vi "个人信息查询跳出界面.vi"() -> (11 "Boolean":bool)   [LabVIEW 2023]
uses:
  <vilib>/Utility/file.llb/Read From Spreadsheet File (string).vi
panel:
  in  "信息查询":i32(listbox)
  in  "输入选项":i32(ring) items=["姓名", "学号", "寝室号"]
  out "Array":string[][](array[string])
  in  "确认":bool
  in  "退出":bool
  in  "姓名/学号/寝室号":string
  # "个人信息查询"
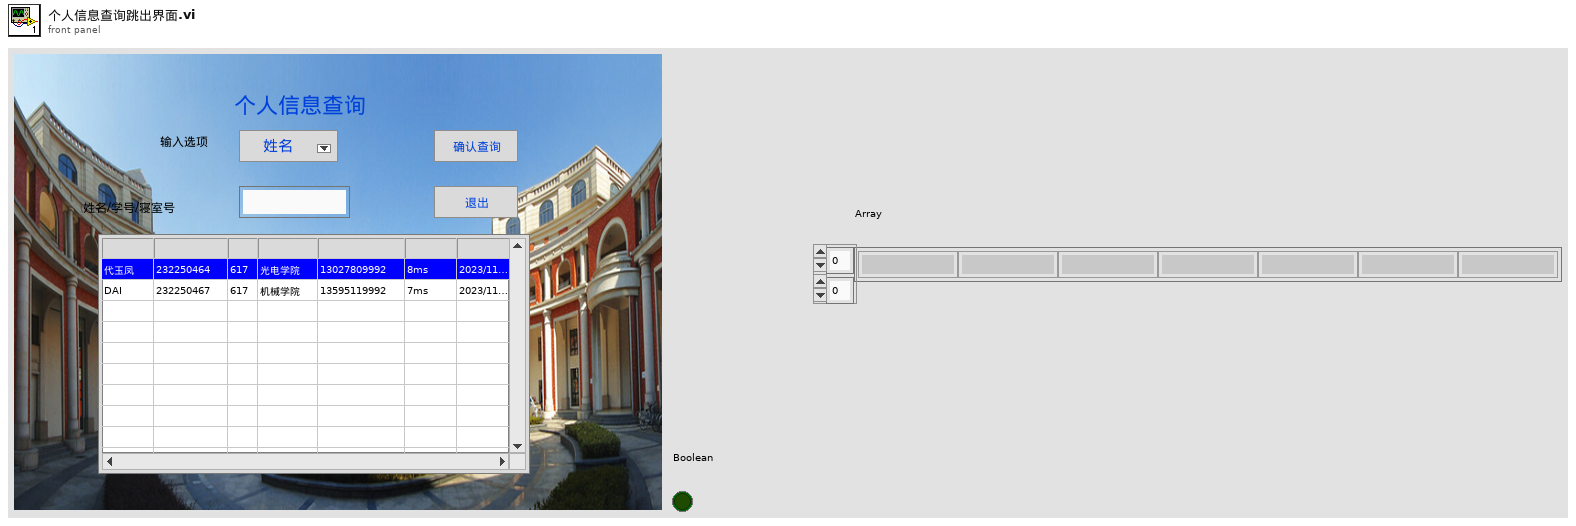
[diagram p1: front panel]
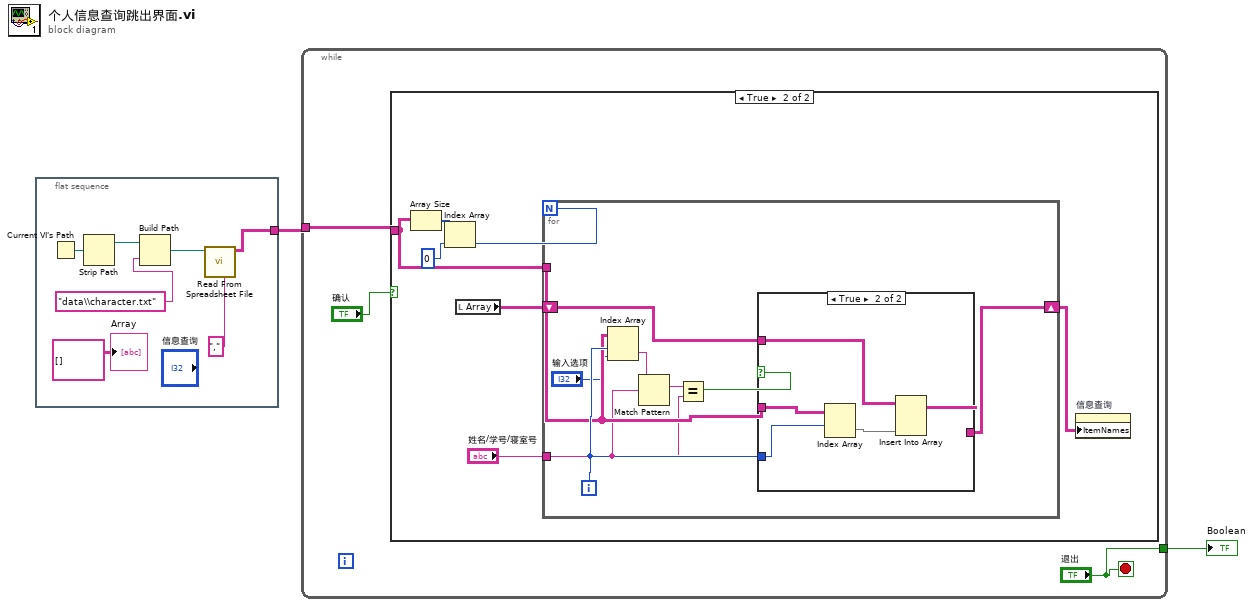
[diagram p0: block diagram]
diagram:
  n1 = flat-sequence {
    tunnel: [w4] -> w2
    frame #0 {
      n2 = Current VI's Path() -> (path=w7:path)
      n3 = Strip Path(path=w7) -> (stripped path=w9:path)  [unwired: 1 out]
      n4 = Build Path(base path=w9, name or relative path="data\\character.txt") -> (appended path=w8:path)
      n5 = call-poly <vilib>:"Read From Spreadsheet File.vi"("delimiter (\\t)"=",", "file path (dialog if empty)"=w8) -> ("all rows"=w4:string[][])  [unwired: 5 in, 4 out]
      "Array" <- string[][] [] ("Array")
    }
  }
  n6 = while {
    tunnel: w2 -> [w11]
    tunnel: ["退出"] -> w1
    stop <- "退出" stop-if-true
    n7 = case shown="True" "确认" {
      tunnel: w11 -> [_ w19]
      frame False {
      }
      frame True {
        n8 = Array Size(array=w19) -> (size(s)=w18:i32[])
        n9 = Index Array(array=w18, index=0) -> (element=w16:i32)
        n10 = local read "Array"() -> (w14:string[][])
        n11 = for {
          N: w16 -> [_]
          tunnel: w19 -> [w26]
          tunnel: "姓名/学号/寝室号" -> [w23]
          shift-right: [w20] -> w13
          shift-left: w14 -> [w21]
          i -> [w27]
          n12 = Index Array(array=w26, index (row)=w27, index (col)="输入选项") -> (element=w24:string)
          n13 = Match Pattern(string=w24, regular expression=w23) -> (match substring=w22:string)  [unwired: 1 in, 3 out]
          n14 = Equal?(x=w22, y=w23) -> (x = y?=w28:bool)
          n15 = case shown="True" w28 {
            tunnel: w27 -> [_ w34]
            tunnel: w26 -> [_ w33]
            tunnel: w21 -> [w29 w31]
            tunnel: [w29 w30] -> w20
            frame False {
            }
            frame True {
              n16 = Index Array(array=w33, index (row)=w34) -> (element=w32:string[])  [unwired: 1 in]
              n17 = Insert Into Array(array=w31, new element=w32) -> (w30:string[][])  [unwired: 2 in]
            }
          }
        }
        n18 = property on="信息查询" class="MCListbox (strict)"("ItemNames"=w13) -> ()  [unwired: 2 in, 2 out]
      }
    }
  }
  "Boolean" <- w1
